vi "Write Message.vi"(6 "timeout ms (25000)":i32, 8 "error in (no error)":errorcluster, 10 "Message":variant, 11 "GenNet Variant Protocol in":refnum<class "GenNet Variant Protocol.lvclass">) -> (0 "error out":errorcluster, 3 "GenNet Variant Protocol out":refnum<class "GenNet Variant Protocol.lvclass">)   [LabVIEW 2022 SP3, in "hse-gennet.lvlib" / "GenNet Variant Protocol.lvclass"]
doc: "____\nHAMPEL SOFTWARE ENGINEERING v3.8.0 (2023-12-18 14:41)"
uses:
  GenNet Variant Protocol.lvclass
  C:/Projects/579-Intelligent-Systems-Term-Project/06_Source/UI/FReVSys_Source/Libraries/hse-libraries/Source/hse-gennet/GenNet Protocols/GenNet Protocol.lvclass
  GenNet Protocol.lvclass/GenNet Protocol.ctl
  Get Connection ID.vi
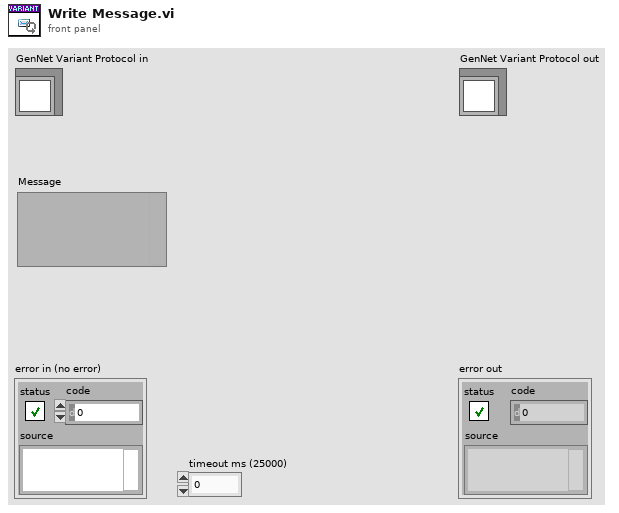
[diagram p1: front panel]
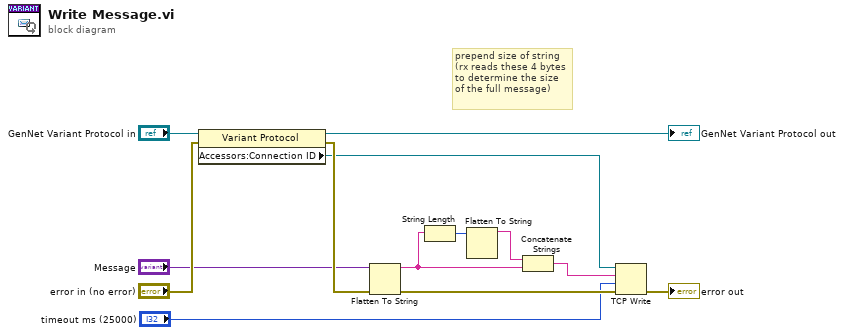
[diagram p0: block diagram]
diagram:
  # "prepend size of string\n(rx reads these 4 bytes\nto determine the size\nof the full message)"
  n1 = property class="Variant Protocol"(reference="GenNet Variant Protocol in", error in="error in (no error)") -> (reference out=→"GenNet Variant Protocol out":refnum<class "GenNet Variant Protocol.lvclass">, error out=w12:errorcluster, "Accessors:Connection ID"=w4:refnum<k5>)
  n2 = Flatten To String(anything="Message", error in (no error)=w12) -> (data string=w5:string, error out=w6:errorcluster)  [unwired: 2 in, 1 out]
  n3 = String Length(string=w5) -> (length=w7:i32)
  n4 = Flatten To String(anything=w7) -> (data string=w8:string)  [unwired: 3 in, 2 out]
  n5 = Concatenate Strings(w8, w5) -> (w9:string)
  n6 = TCP Write(connection ID=w4, data in=w9, error in (no error)=w6, 9:"timeout ms (25000)") -> (error out=→"error out":errorcluster)  [unwired: 2 out]
